vi "Micro-PL v10.2.0.vi"() -> ()   [LabVIEW 2010]
uses:
  drivers/Oxford ITC/ITCAPPS.LLB/ITCSetup.ctl
  drivers/Oxford ITC/ITCSUBS.LLB/ITCIO.ctl
  drivers/Oxford ITC/BUSGEN.LLB/OxfordAddress.ctl
  drivers/Oxford ITC/ITCSUBS.LLB/ITCVersion.ctl
  subvi/ESA-C/TypeDefs/ESA-C Live Controls.ctl
  subvi/ESA-C/TypeDefs/ESA-C Current Values.ctl
  subvi/ESA-C/TypeDefs/ESA-C Connection Settings.ctl
  subvi/ESA-C/TypeDefs/ESA-C Set Positions.ctl
  subvi/ITC503/TypeDefs/ITC503 Settings.ctl
  subvi/ITC503/TypeDefs/ITC503 Current Values.ctl
  subvi/iHR550/TypeDefs/iHR Current Values.ctl
  subvi/iHR550/TypeDefs/iHR Settings.ctl
  subvi/Mapping/TypeDefs/Mapping Spectra Params.ctl
  <vilib>/Utility/miscctls.llb/LVBoundsTypeDef.ctl
  <vilib>/Utility/miscctls.llb/LVPointTypeDef.ctl
  drivers/Horiba Spectrum One 3000V/Lib/CCD_command.llb/Comm Params.ctl
panel:
  out "ITC503 Temp Storage":dbl
  out "Runtime":u32
  out "ITC Gradient Time":i64
  out "Read ITC":bool
  out "Read CCD3500":bool
  out "Read iHR550":bool
  out "Read Drive":bool
  out "Spectrum Properties":cluster{"Position":T1, "Plot Area Size":T1}={"Position"={"Width"=36, "Height"=367}, "Plot Area Size"={"Width"=496, "Height"=264}}
  in  "Auto Folder":path caption="Ausgewählter Pfad"
  out "Int. Time Temp":dbl
  out "Wavelengths (nm)":dbl[](array[numeric])
  out "Measurement Running":bool
  out "ITC503s Running":bool
  out "Drive Running":bool
  out "CCD3500V Running":bool
  out "iHR550 Running":bool
  in  "Exit":bool
  out "iHR550 Status":bool
  out "Drive Status":bool
  out "CCD3500V Status":bool
  out "ITC503 Status":bool
  in  "CCD3500V Connection":T2={"Comm Interface"=1, "BUS"=0, "Address"=5, "Com Port"=0}
  out "Video Running":bool
  out "iHR550 RefNum":refnum<k7> caption="Mono RefNum out"
  out "ITC Setup":T3={"Description"="", "IO Info"={"Address"={"Com Port"=1, "ISOBUS Address"=1, "GPIB Address"=24, "Communication"=enum."ISOBUS"}, "Version"=enum."ITC503", "Ch 1 dec places"=1, "Ch 2 dec places"=1, "Ch 3 dec places"=1, "Ch1 Name"="", "Ch2 Name"="", "Ch3 Name"=""}}
  in  "Register":enum32{"Devices", "Acquisition / Mapping"}(tab)
  out "CCD3500 Temperature":dbl caption="Temp. (°C)" min=10.0 max=160.0 step=0.1 format="%.1f"
  in  "CCD3500V GPIB-Port":i32=5 caption="GPIB-Port" min=1 max=20 step=1 format="%#.0f"
  in  "CCD3500V Connect":bool
  out "CCD Timing":u32 caption="CCD"
  out "ITC Timing":u32 caption="ITC"
  out "Drive Timing":u32 caption="Drive"
  out "iHR550 Timing":u32 caption="iHR550"
  in  "iHR550 Force Init":bool=TRUE
  in  "iHR550 Connect":bool
  in  "iHR550 ID":string(combo)="iHR550" caption="Monochromator ID"
  out "ITC503 Current Values":T7 {"ITC503 Gradient" format="%.2f"; "ITC503 Setpoint" min=-273.0 max=300000.0 step=0.0001 format="%.1f"; "ITC503 I" format="%_1f"; "ITC503 P" format="%_1f"; "ITC503 Temperature" min=0.0 max=1645.0 step=1e-05 format="%.2f"; "ITC503 Heater" min=0.0 max=100.0 step=0.01 scale=0.0..100.0}
  in  "ITC503 Settings":T8={"ITC503 Set Setpoint"=0.0, "ITC503 Set Auto Heater"=TRUE, "ITC503 Set Auto PID"=TRUE, "P"=0.0, "I"=0.0, "D"=0.0} {"D" min=0.0 max=100.0 step=0.1 format="%.1f"; "I" min=0.0 max=100.0 step=0.1 format="%.1f"; "P" min=0.0 max=100.0 step=0.1 format="%.1f"; "ITC503 Set Setpoint" min=-273.0 max=300000.0 step=0.1 format="%.1f"}
  in  "ITC503 Configure":bool
  in  "ITC503 Connect":bool
  in  "ITC503 Selector":u16(ring) caption="Select Device" items=["ITC503s"]
  out "Drive Current Values":T9 {"Position"."Drive Z Position" min=-273.0 max=300000.0 step=0.0001 format="%.1f"; "Position"."Drive Y Position" min=-273.0 max=300000.0 step=0.0001 format="%.1f"; "Position"."Drive X Position" min=-273.0 max=300000.0 step=0.0001 format="%.1f"; "Voltages"."Drive Z Voltage" min=-273.0 max=300000.0 step=0.0001 format="%.1f"; "Voltages"."Drive Y Voltage" min=-273.0 max=300000.0 step=0.0001 format="%.1f"; "Voltages"."Drive X Voltage" min=-273.0 max=300000.0 step=0.0001 format="%.1f"}
  in  "Drive Connection":T10={"Objective GPIB-Port"=4, "Stage GPIB-Port"=4, "Drive Selector"=0, "Drive Velocity (V/s)"=5.0} {"Drive Velocity (V/s)" min=10.0 max=160.0 step=0.1 format="%.1f"; "Drive Selector" items=["Obj.", "Stage"]; "Stage GPIB-Port" min=1 max=20 step=1 format="%#.0f"; "Objective GPIB-Port" min=1 max=20 step=1 format="%#.0f"}
  in  "Drive Connect":bool
  in  "Spectrum Maximize":bool
  out "Spectrum":cluster{dbl[], dbl[]}[](graph)
  in  "CCD3000 Current Rep.":string="0/0"
  in  "Spectrum Load":bool
  in  "Spectrum Save":bool
  in  "Video Show":bool
  in  "Drive GoTo":bool caption="Objective Move Abs."
  in  "Drive New Positions":T11 {"Drive X Set" min=10.0 max=160.0 step=0.1 format="%.1f"; "Drive Z Set" min=10.0 max=160.0 step=0.1 format="%.1f"; "Drive Y Set" min=10.0 max=160.0 step=0.1 format="%.1f"}
  in  "Spectrum Autosave":bool caption="iHR550 Force Init"
  in  "CCD3500 Preview":bool
  in  "CCD3500 Acquire":bool
  in  "Spectra Settings":T12={"Integration Time"=1.0, "Repetitions"=1, "Mapping Spectra"=TRUE} caption="Mapping Spectra Settings" {"Repetitions" min=1 max=100 step=1; "Integration Time" min=0.1 max=6000.0 step=0.1 format="%.1f"}
  in  "Mapping Start":bool
  in  "iHR550 Configure":bool
  in  "iHR Settings":T13={"iHR550 Set Exit Mirror"=2, "iHR550 Set Side Exit"=0.0, "iHR550 Set Front Entrance"=0.0, "iHR550 Set Wavelength"=897.9988, "iHR550 Set Grating"=0, "iHR550 Set Grating Switch"=FALSE, "iHR550 Set Wavelength Switch"=FALSE, "iHR550 Set Mirror Switch"=FALSE, "iHR550 Set Slits Switch"=FALSE} {"iHR550 Set Grating" items=["1800"=1, "600"=2, "150"=3]; "iHR550 Set Wavelength" min=0.0 max=1500.0 step=1.0; "iHR550 Set Side Exit" min=0.0 max=2000.0 step=1.0; "iHR550 Set Exit Mirror" items=["Front"=2, "Side"=3]}
  out "iHR Current Values":T14={"iHR 550 Front Entrance"=0.0, "iHR550 Side Exit"=0.0, "iHR550 Wavelength"=897.9988, "iHR550 Exit Mirror"=2, "iHR550 Grating"="1", "Grating Index"=1} {"iHR550 Exit Mirror" items=["EntranceMirror", "ExitMirror", "Front", "Side"]}
  out "Drive Live Current Values":T9 {"Position"."Drive Z Position" min=-273.0 max=300000.0 step=0.0001 format="%.1f"; "Position"."Drive Y Position" min=-273.0 max=300000.0 step=0.0001 format="%.1f"; "Position"."Drive X Position" min=-273.0 max=300000.0 step=0.0001 format="%.1f"; "Voltages"."Drive Z Voltage" min=-273.0 max=300000.0 step=0.0001 format="%.1f"; "Voltages"."Drive Y Voltage" min=-273.0 max=300000.0 step=0.0001 format="%.1f"; "Voltages"."Drive X Voltage" min=-273.0 max=300000.0 step=0.0001 format="%.1f"}
  in  "Drive Live Controls":T15={"Snapshot"=FALSE, "Move Step"=1.0, "Move Home"=FALSE, "Move Down"=FALSE, "Move Up"=FALSE, "Move Left"=FALSE, "Move Right"=FALSE, "Move Out"=FALSE, "Move In"=FALSE} {"Move Step" min=0.0 max=30.0 step=0.1 format="%.1f"}
  # "Correlation Setup"
  # "Active"
  # "Active"
  # "ITC"
  # "iHR"
  # "Drive"
  # "CCD"
  # "Status"
  # "CCD"
  # "ITC"
  # "iHR"
  # "Drive"
  # "CCD"
  # "Timing"
  # "Monochromator"
  # "Cryostat"
  # "Drives"
  # "Drive Control"
  # "Spectrum"
  # "CCD"
  # "Mapping"
  # "Launch the Spectral Mapping VI and Raman Tool Set 2.0 in a new window."
  # "Monochromator"
  # "XY"
  # "Z"
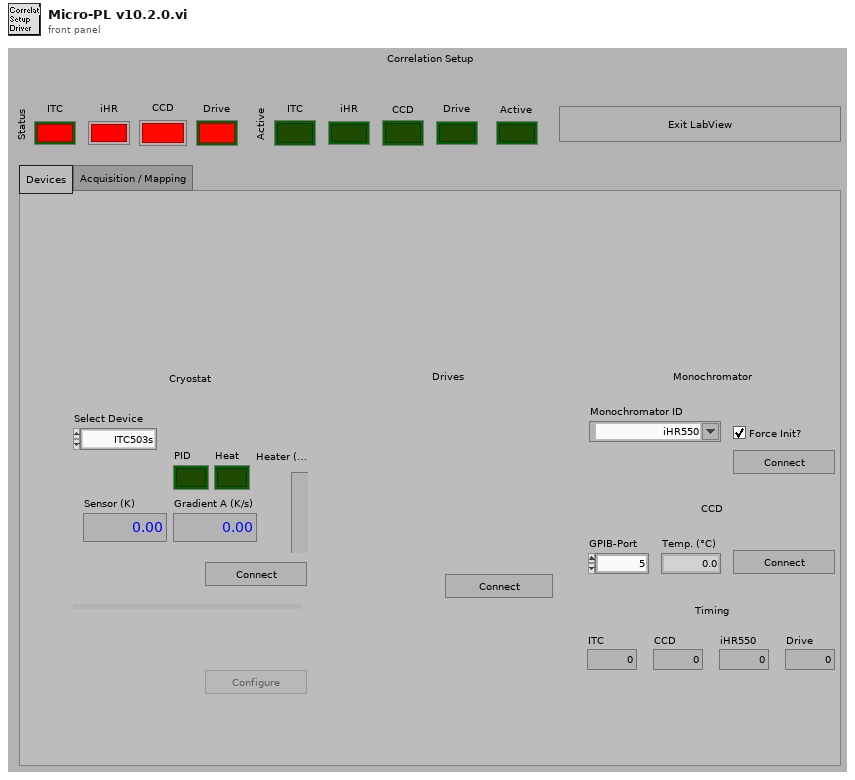
[diagram p1: front panel]
types:
  T1 = typedef "LVBoundsTypeDef.ctl" = cluster{"Width":u32, "Height":u32}
  T2 = cluster{"Comm Interface":u16, "BUS":i16, "Address":i16, "Com Port":i32}
  T3 = typedef "ITCSetup.ctl" = cluster{"Description":string, "IO Info":T4}
  T4 = typedef "ITCIO.ctl" = cluster{"Address":T5, "Version":T6, "Ch 1 dec places":i16, "Ch 2 dec places":i16, "Ch 3 dec places":i16, "Ch1 Name":string, "Ch2 Name":string, "Ch3 Name":string}
  T5 = typedef "OxfordAddress.ctl" = cluster{"Com Port":i32, "ISOBUS Address":i32, "GPIB Address":i16, "Communication":enum16{"RS232", "ISOBUS", "GPIB", "Gateway"}}
  T6 = typedef "ITCVersion.ctl" = enum16{"ITC502", "ITC503", "ITC601"}
  T7 = typedef "ITC503 Current Values.ctl" = cluster{"ITC503 Heater":dbl, "ITC503 Temperature":dbl, "ITC503 P":dbl, "ITC503 I":dbl, "ITC503 D":dbl, "ITC503 Setpoint":dbl, "ITC503 Gradient":dbl, "ITC503 Heater Auto":bool, "ITC503 PID Auto":bool}
  T8 = typedef "ITC503 Settings.ctl" = cluster{"ITC503 Set Setpoint":dbl, "ITC503 Set Auto Heater":bool, "ITC503 Set Auto PID":bool, "P":dbl, "I":dbl, "D":dbl}
  T9 = typedef "ESA-C Current Values.ctl" = cluster{"Voltages":cluster{"Drive X Voltage":dbl, "Drive Y Voltage":dbl, "Drive Z Voltage":dbl}, "Position":cluster{"Drive X Position":dbl, "Drive Y Position":dbl, "Drive Z Position":dbl}}
  T10 = typedef "ESA-C Connection Settings.ctl" = cluster{"Objective GPIB-Port":i32, "Stage GPIB-Port":i32, "Drive Selector":u16, "Drive Velocity (V/s)":dbl}
  T11 = typedef "ESA-C Set Positions.ctl" = cluster{"Drive X Set":dbl, "Drive Y Set":dbl, "Drive Z Set":dbl}
  T12 = typedef "Mapping Spectra Params.ctl" = cluster{"Integration Time":dbl, "Repetitions":u16, "Mapping Spectra":bool}
  T13 = typedef "iHR Settings.ctl" = cluster{"iHR550 Set Exit Mirror":u16, "iHR550 Set Side Exit":dbl, "iHR550 Set Front Entrance":dbl, "iHR550 Set Wavelength":dbl, "iHR550 Set Grating":u16, "iHR550 Set Grating Switch":bool, "iHR550 Set Wavelength Switch":bool, "iHR550 Set Mirror Switch":bool, "iHR550 Set Slits Switch":bool}
  T14 = typedef "iHR Current Values.ctl" = cluster{"iHR 550 Front Entrance":dbl, "iHR550 Side Exit":dbl, "iHR550 Wavelength":dbl, "iHR550 Exit Mirror":i32, "iHR550 Grating":string, "Grating Index":i32}
  T15 = typedef "ESA-C Live Controls.ctl" = cluster{"Snapshot":bool, "Move Step":dbl, "Move Home":bool, "Move Down":bool, "Move Up":bool, "Move Left":bool, "Move Right":bool, "Move Out":bool, "Move In":bool}
  T16 = typedef "LVPointTypeDef.ctl" = cluster{"Horizontal":i16, "Vertical":i16}
  T17 = enum8{"Enabled", "Disabled", "Disabled and Grayed Out"}
  T18 = typedef "Comm Params.ctl" = cluster{"Comm Interface":u16, "BUS":i16, "Address":i16, "Com Port":i32}
  T19 = enum16{"CCD Temperature Z345", "CCD Temperature Z308", "CCD Gain"}
  T20 = cluster{"CCD3000 Connection":T18, "Drive Connection Settings":T10, "ITC503 Current Values":T7, "Wavelengths (nm)":dbl[], "Drive Current Values":T9, "iHR Current Values":T14, "Spectra Settings":T12, "CCD3500 Temperature":dbl, "Simulate Drive 2":bool, "Simulate Spectra 2":bool}
  T21 = cluster{"Intensities":dbl[], "Wavelengths":dbl[]}[]
  T22 = typedef "LVPositionTypeDef.ctl" = cluster{"Left":i32, "Top":i32}
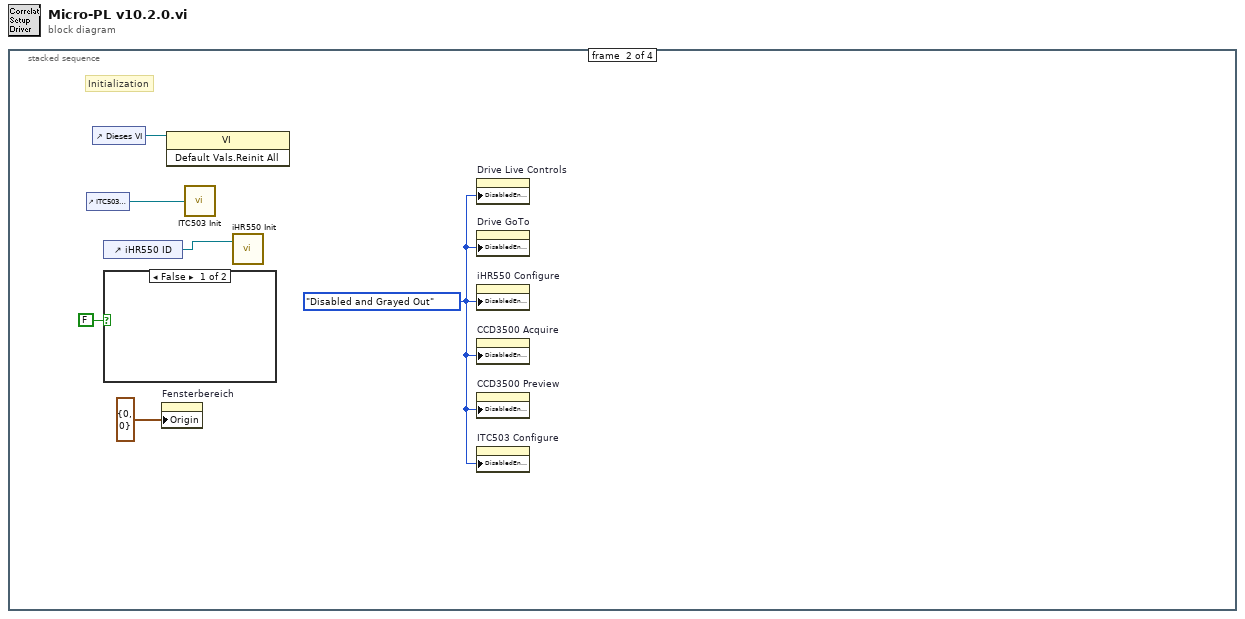
[diagram p0: block diagram]
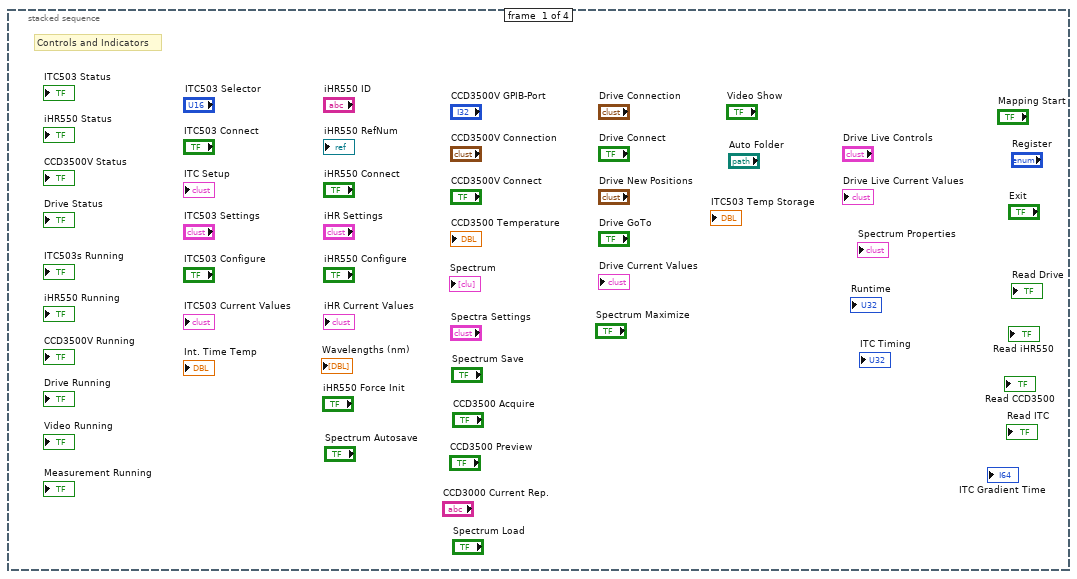
[diagram p2: hidden frame]
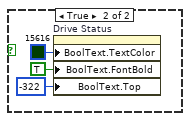
[diagram p3: hidden frame]
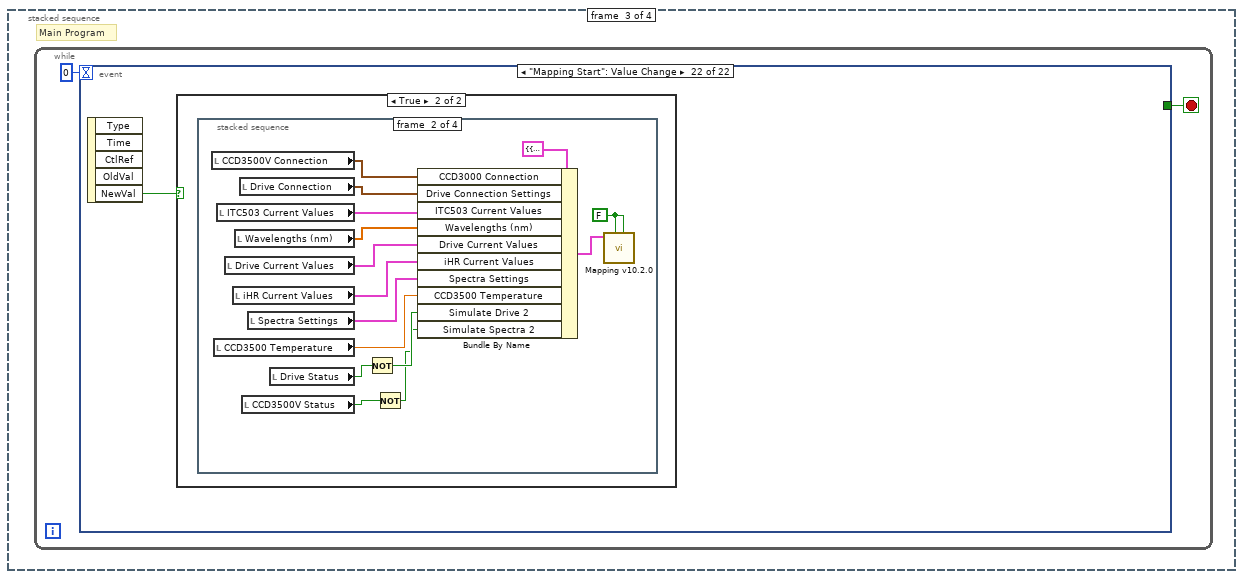
[diagram p4: hidden frame]
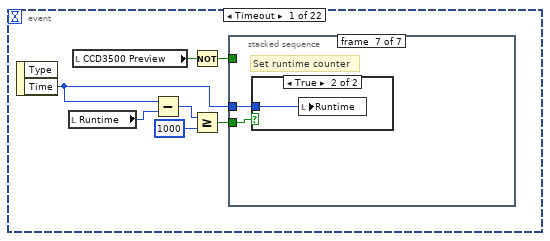
[diagram p5: hidden frame]
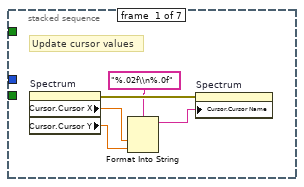
[diagram p6: hidden frame]
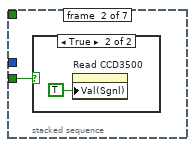
[diagram p7: hidden frame]
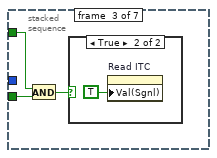
[diagram p9: hidden frame]
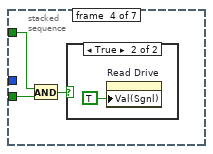
[diagram p11: hidden frame]
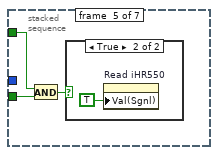
[diagram p13: hidden frame]
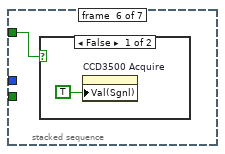
[diagram p15: hidden frame]
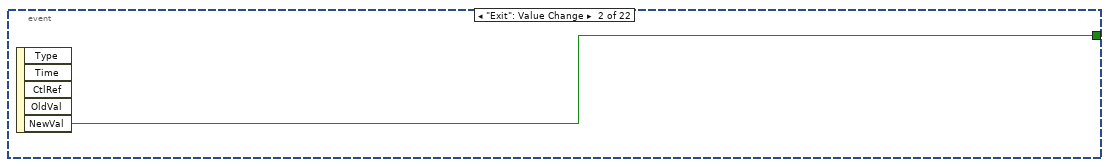
[diagram p18: hidden frame]
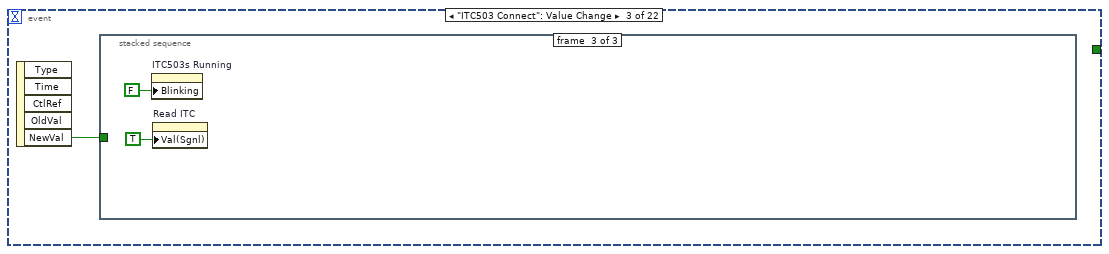
[diagram p19: hidden frame]
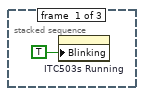
[diagram p20: hidden frame]
diagram:
  n1 = stacked-sequence {
    frame #0 {
      # "Controls and Indicators"
    }
    frame #1 {
      w1 = T17."Disabled and Grayed Out" ("Deaktiviert")
      # "Initialization"
      n2 = control-ref of="ITC503 Selector"() -> (w6:refnum<vi>)
      n3 = control-ref of="Dieses VI"() -> (w5:refnum<vi>)
      n4 = control-ref of="iHR550 ID"() -> (w4:refnum<vi>)
      n5 = case shown="False" FALSE {
        frame False {
        }
        frame True {
          n6 = property on="Drive Status" class="Bool (strict)"("BoolText.TextColor"=u32 15616, "BoolText.FontBold"=TRUE ("Boolescher Text.Schriftart:Fett"), "BoolText.Top"=-322 ("Boolescher Text.Position:Oben")) -> ()  [unwired: 2 in, 2 out]
        }
      }
      n7 = property on="Fensterbereich" class="Pane"("Origin"=T16 {"Horizontal"=0, "Vertical"=0}) -> ()  [unwired: 2 in, 2 out]
      n8 = invoke class="VI" method="Default Vals.Reinit All"(reference=w5) -> ()  [unwired: 2 in, 3 out]
      n9 = call "ITC503 Init.vi"("ITC Selector"=w6) -> ()  [unwired: 1 in]
      n10 = call "iHR550 Init.vi"("Mono ID"=w4) -> ()  [unwired: 2 in]
      n11 = property on="Drive Live Controls" class="Clust (strict)"("DisabledEnum"=w1) -> ()  [unwired: 2 in, 2 out]
      n12 = property on="Drive GoTo" class="Bool (strict)"("DisabledEnum"=w1) -> ()  [unwired: 2 in, 2 out]
      n13 = property on="iHR550 Configure" class="Bool (strict)"("DisabledEnum"=w1) -> ()  [unwired: 2 in, 2 out]
      n14 = property on="CCD3500 Acquire" class="Bool (strict)"("DisabledEnum"=w1) -> ()  [unwired: 2 in, 2 out]
      n15 = property on="CCD3500 Preview" class="Bool (strict)"("DisabledEnum"=w1) -> ()  [unwired: 2 in, 2 out]
      n16 = property on="ITC503 Configure" class="Bool (strict)"("DisabledEnum"=w1) -> ()  [unwired: 2 in, 2 out]
    }
    frame #2 {
      # "Main Program"
      n17 = while "Main-Program" {
        stop <- w11 stop-if-true
        n18 = event shown="[21] \"Mapping Start\": Value Change" {
          selector: _ -> [_ _ _ _ _ _ _ _ _ _ _ _ _ _ _ _ _ _ _ _ _ _]
          dyn-events: _ -> [_ _ _ _ _ _ _ _ _ _ _ _ _ _ _ _ _ _ _ _ _ _]
          timeout: 0 -> [_ _ _ _ _ _ _ _ _ _ _ _ _ _ _ _ _ _ _ _ _ _]
          tunnel: [_ w43 _ _ _ _ _ _ _ _ _ _ _ _ _ _ _ _ _ _ _ _] -> w11
          event Timeout {
            n19 = event-data() -> ("Time"=w13:u32)  [unwired: 1 in, 1 out]
            n20 = local read "Runtime"() -> (w12:u32)
            n21 = local read "CCD3500 Preview"() -> (w15:bool)
            n22 = Subtract(x=w13, y=w12) -> (x-y=w16:u32)
            n23 = Not(x=w15) -> (.not. x?=w14:bool)
            n24 = Greater Or Equal?(x=w16, y=u32 1000) -> (x >= y?=w17:bool)
            n25 = stacked-sequence {
              tunnel: w17 -> [_ w24 w28 w32 w36 _ w40]
              tunnel: w13 -> [_ _ _ _ _ _ w41]
              tunnel: w14 -> [_ _ w27 w31 w35 w38 _]
              frame #0 {
                # "Update cursor values"
                n26 = property on="Spectrum" class="XYGraph (strict)"() -> (error out=w23:errorcluster, "Cursor.Cursor X"=w22:dbl, "Cursor.Cursor Y"=w21:dbl)  [unwired: 2 in, 1 out]
                n27 = Format Into String(format string="%.02f\\n%.0f", w22, w21) -> (resulting string=w19:string)  [unwired: 2 in, 1 out]
                n28 = property on="Spectrum" class="XYGraph (strict)"(error in=w23, "Cursor.Cursor Name"=w19) -> ()  [unwired: 1 in, 2 out]
              }
              frame #1 {
                n29 = case shown="True" w24 {
                  frame False {
                  }
                  frame True {
                    n30 = property on="Read CCD3500" class="Bool (strict)"("Val(Sgnl)"=TRUE ("Value (Signaling)")) -> ()  [unwired: 2 in, 2 out]
                  }
                }
              }
              frame #2 {
                n31 = And(x=w27, y=w28) -> (x .and. y?=w26:bool)
                n32 = case shown="True" w26 {
                  frame False {
                  }
                  frame True {
                    n33 = property on="Read ITC" class="Bool (strict)"("Val(Sgnl)"=TRUE ("Value (Signaling)")) -> ()  [unwired: 2 in, 2 out]
                  }
                }
              }
              frame #3 {
                n34 = And(x=w31, y=w32) -> (x .and. y?=w30:bool)
                n35 = case shown="True" w30 {
                  frame False {
                  }
                  frame True {
                    n36 = property on="Read Drive" class="Bool (strict)"("Val(Sgnl)"=TRUE ("Value (Signaling)")) -> ()  [unwired: 2 in, 2 out]
                  }
                }
              }
              frame #4 {
                n37 = And(x=w35, y=w36) -> (x .and. y?=w34:bool)
                n38 = case shown="True" w34 {
                  frame False {
                  }
                  frame True {
                    n39 = property on="Read iHR550" class="Bool (strict)"("Val(Sgnl)"=TRUE ("Value (Signaling)")) -> ()  [unwired: 2 in, 2 out]
                  }
                }
              }
              frame #5 {
                n40 = case shown="False" w38 {
                  frame False {
                    n41 = property on="CCD3500 Acquire" class="Bool (strict)"("Val(Sgnl)"=TRUE ("Wert (signalisierend)")) -> ()  [unwired: 2 in, 2 out]
                  }
                  frame True {
                  }
                }
              }
              frame #6 {
                # "Set runtime counter"
                n42 = case shown="True" w40 {
                  tunnel: w41 -> [_ w42]
                  frame False {
                  }
                  frame True {
                    n43 = local write "Runtime"(w42) -> ()
                  }
                }
              }
            }
          }
          event "Exit": Value Change {
            n44 = event-data() -> ("NewVal"=w43:bool)  [unwired: 1 in, 4 out]
          }
          event "ITC503 Connect": Value Change {
            n45 = event-data() -> ("NewVal"=w44:bool)  [unwired: 1 in, 4 out]
            n46 = stacked-sequence {
              tunnel: w44 -> [_ w46 _]
              frame #0 {
                n47 = property on="ITC503s Running" class="Bool (strict)"("Blinking"=TRUE ("Blinkend")) -> ()  [unwired: 2 in, 2 out]
              }
              frame #1 {
                n48 = case shown="True" w46 {
                  selector: w46 -> [w51 _]
                  tunnel: [w51 w58] -> w48
                  frame False {
                    # "disconnect"
                    n49 = control-ref of="ITC503s Running"() -> (w52:refnum<vi>)
                    n50 = property class="Bool (strict)"(reference=w52, "Blinking"=w51, "Value"=w51) -> ()  [unwired: 1 in, 2 out]
                  }
                  frame True {
                    # "connect"
                    n51 = local read "ITC503 Selector"() -> (w59:u16)
                    n52 = call "ITC503 Connect.vi"("ITC Selector"=w59) -> ("ITC Setup"=w57:T3, "Connected"=w58:bool)
                    n53 = local write "ITC Setup"(w57) -> ()
                    n54 = call "ITC503 Get Values.vi"("ITC Setup"=w57) -> ("ITC503 Current Values"=w56:T7)  [unwired: 1 in, 1 out]
                    n55 = Unbundle By Name(w56) -> ("ITC503 Setpoint"=w53:dbl)
                    n56 = Bundle By Name(cluster=T8 {"ITC503 Set Setpoint"=0.0, "ITC503 Set Auto Heater"=TRUE, "ITC503 Set Auto PID"=TRUE, "P"=0.0, "I"=0.0, "D"=0.0} ("ITC503 Settings"), "ITC503 Set Setpoint"=w53) -> (w54:T8)
                    n57 = local write "ITC503 Settings"(w54) -> ()
                  }
                }
                n58 = case shown="False" w48 {
                  tunnel: [T17."Disabled and Grayed Out" ("Deaktiviert") T17."Enabled" ("Deaktiviert")] -> w47
                  frame False {
                  }
                  frame True {
                  }
                }
                n59 = local write "ITC503 Status"(w48) -> ()
                n60 = local write "ITC503 Connect"(w48) -> ()
                n61 = property on="ITC503 Configure" class="Bool (strict)"("DisabledEnum"=w47) -> ()  [unwired: 2 in, 2 out]
              }
              frame #2 {
                n62 = property on="ITC503s Running" class="Bool (strict)"("Blinking"=FALSE ("Blinkend")) -> ()  [unwired: 2 in, 2 out]
                n63 = property on="Read ITC" class="Bool (strict)"("Val(Sgnl)"=TRUE ("Wert (signalisierend)")) -> ()  [unwired: 2 in, 2 out]
              }
            }
          }
          event "Read ITC": Value Change {
            n64 = event-data() -> ("Time"=w63:u32, "NewVal"=w67:bool)  [unwired: 1 in, 3 out]
            n65 = local read "ITC503 Status"() -> (w66:bool)
            n66 = control-ref of="ITC503s Running"() -> (w64:refnum<vi>)
            n67 = And(x=w66, y=w67) -> (x .and. y?=w65:bool)
            n68 = case shown="True" w65 {
              tunnel: w64 -> [w69 w73]
              tunnel: w63 -> [_ w72]
              tunnel: [u32 0 w71] -> w62
              frame False {
                n69 = property class="Bool (strict)"(reference=w69, "BoolText.Text"="" ("Boolescher Text.Text")) -> ()  [unwired: 1 in, 2 out]
              }
              frame True {
                n70 = stacked-sequence {
                  seq-local: [_ w78 _ _] -> [_ _ w95 _]
                  seq-local: [w74 _ _ _] -> [_ _ _ w101]
                  tunnel: w73 -> [_ _ w88 _]
                  tunnel: w72 -> [_ w79 _ _]
                  tunnel: [_ _ _ w102] -> w71
                  frame #0 {
                    n71 = Tick Count (ms)() -> (millisecond timer value=w74:u32)
                  }
                  frame #1 {
                    n72 = local read "ITC Setup"() -> (w86:T3)
                    n73 = local read "ITC Gradient Time"() -> (w83:i64)
                    n74 = call "ITC503 Get Values.vi"("ITC Setup"=w86) -> ("ITC503 Current Values"=w78:T7)  [unwired: 1 in, 1 out]
                    n75 = local read "ITC503 Temp Storage"() -> (w77:dbl)
                    n76 = Unbundle By Name(w78) -> ("ITC503 Temperature"=w75:dbl)
                    n77 = Subtract(x=w79, y=w83) -> (x-y=w82:i64)
                    n78 = Divide(x=w82, y=i64 1000) -> (x/y=w80:dbl)
                    n79 = Subtract(x=w75, y=w77) -> (x-y=w76:dbl)
                    n80 = Divide(x=w76, y=w80) -> (x/y=w85:dbl)
                    n81 = Bundle By Name(cluster=w78, "ITC503 Gradient"=w85) -> (w84:T7)
                    n82 = local write "ITC503 Current Values"(w84) -> ()
                  }
                  frame #2 {
                    n83 = Unbundle By Name(w95) -> ("ITC503 Temperature"=w87:dbl, "ITC503 Setpoint"=w96:dbl)
                    n84 = Subtract(x=w87, y=w96) -> (x-y=w97:dbl)
                    n85 = Number To Fractional String(number=w87, precision (6)=i16 2 ("Genauigkeit (6)")) -> (F-format string=w91:string)  [unwired: 2 in]
                    n86 = Absolute Value(x=w97) -> (abs(x)=w98:dbl)
                    n87 = String Subset(string=w91, length (rest)=5 ("Länge (Rest)")) -> (substring=w89:string)  [unwired: 1 in]
                    n88 = Greater?(x=w98, y=2.0) -> (0:w94:bool)
                    n89 = Not(x=w94) -> (.not. x?=w93:bool)
                    n90 = property class="Bool (strict)"(reference=w88, "Blinking"=w94, "Value"=w93, "BoolText.Text"=w89) -> ()  [unwired: 1 in, 2 out]
                    n91 = local write "ITC503 Temp Storage"(w87) -> ()
                  }
                  frame #3 {
                    n92 = Tick Count (ms)() -> (millisecond timer value=w100:u32)
                    n93 = local write "ITC Gradient Time"(w100) -> ()
                    n94 = Subtract(x=w100, y=w101) -> (x-y=w102:u32)
                  }
                }
              }
            }
            n95 = local write "ITC Timing"(w62) -> ()
          }
          event "iHR550 Connect": Value Change {
            n96 = event-data() -> ("NewVal"=w103:bool)  [unwired: 1 in, 4 out]
            n97 = stacked-sequence {
              tunnel: w103 -> [_ w106 _]
              frame #0 {
                n98 = property on="iHR550 Running" class="Bool (strict)"("Blinking"=TRUE ("Blinkend")) -> ()  [unwired: 2 in, 2 out]
              }
              frame #1 {
                n99 = case shown="True" w106 {
                  selector: w106 -> [w110 _]
                  tunnel: [w110 w123] -> w105
                  frame False {
                    # "disconnect"
                  }
                  frame True {
                    # "connect"
                    n100 = local read "iHR550 Force Init"() -> (w121:bool)
                    n101 = control-ref of="iHR550 Set Grating"() -> (w122:refnum<vi>)
                    n102 = local read "iHR550 ID"() -> (w124:string)
                    n103 = call "iHR550 Connect.vi"("Force\nInitialization"=w121, "Grating Selector"=w122, "Mono ID"=w124) -> ("Initialized"=w123:bool, "iHR550 RefNum"=w120:refnum<k7>)  [unwired: 2 in, 4 out]
                    n104 = local write "iHR550 RefNum"(w120) -> ()
                    n105 = call "iHR550 Read Values.vi"("JYMONOLib.IJYMonoReqd"=w120) -> ("iHR Current Values"=w112:T14)  [unwired: 1 in]
                    n106 = local write "iHR Current Values"(w112) -> ()
                    n107 = Unbundle By Name(w112) -> ("iHR 550 Front Entrance"=w118:dbl, "iHR550 Side Exit"=w117:dbl, "iHR550 Wavelength"=w116:dbl, "iHR550 Exit Mirror"=w115:i32, "Grating Index"=w113:i32)
                    n108 = call "iHR550 Convert Axis.vi"("iHR Current Values"=w112) -> ("Wavelengths (nm)"=w111:dbl[])
                    n109 = local write "Wavelengths (nm)"(w111) -> ()
                    n110 = Bundle By Name(cluster=T13 {"iHR550 Set Exit Mirror"=0, "iHR550 Set Side Exit"=0.0, "iHR550 Set Front Entrance"=0.0, "iHR550 Set Wavelength"=0.0, "iHR550 Set Grating"=0, "iHR550 Set Grating Switch"=FALSE, "iHR550 Set Wavelength Switch"=FALSE, "iHR550 Set Mirror Switch"=FALSE, "iHR550 Set Slits Switch"=FALSE} ("iHR Settings"), "iHR550 Set Front Entrance"=w118, "iHR550 Set Side Exit"=w117, "iHR550 Set Wavelength"=w116, "iHR550 Set Exit Mirror"=w115, "iHR550 Set Grating"=w113) -> (w114:T13)
                    n111 = local write "iHR Settings"(w114) -> ()
                  }
                }
                n112 = local write "iHR550 Status"(w105) -> ()
                n113 = local write "iHR550 Connect"(w105) -> ()
                n114 = case shown="False" w105 {
                  tunnel: [T17."Disabled and Grayed Out" ("Deaktiviert") T17."Enabled" ("Deaktiviert")] -> w107
                  frame False {
                  }
                  frame True {
                  }
                }
                n115 = property on="iHR550 Configure" class="Bool (strict)"("DisabledEnum"=w107) -> ()  [unwired: 2 in, 2 out]
              }
              frame #2 {
                n116 = local write "iHR550 Force Init"(FALSE ("iHR550 Force Init")) -> ()
                n117 = property on="iHR550 Running" class="Bool (strict)"("Blinking"=FALSE ("Blinkend")) -> ()  [unwired: 2 in, 2 out]
                n118 = property on="Read iHR550" class="Bool (strict)"("Val(Sgnl)"=TRUE ("Wert (signalisierend)")) -> ()  [unwired: 2 in, 2 out]
              }
            }
          }
          event "Read iHR550": Value Change {
            n119 = event-data() -> ("NewVal"=w131:bool)  [unwired: 1 in, 4 out]
            n120 = local read "iHR550 Status"() -> (w130:bool)
            n121 = And(x=w130, y=w131) -> (x .and. y?=w129:bool)
            n122 = case shown="False" w129 {
              tunnel: [u32 0 w133] -> w128
              frame False {
              }
              frame True {
                n123 = stacked-sequence {
                  seq-local: [w134 _ _] -> [_ _ w137]
                  tunnel: [_ _ w138] -> w133
                  frame #0 {
                    n124 = Tick Count (ms)() -> (millisecond timer value=w134:u32)
                  }
                  frame #1 {
                    n125 = local read "iHR550 RefNum"() -> (w136:refnum<k7>)
                    n126 = call "iHR550 Read Values.vi"("JYMONOLib.IJYMonoReqd"=w136) -> ("iHR Current Values"=w135:T14)  [unwired: 1 in]
                    n127 = local write "iHR Current Values"(w135) -> ()
                  }
                  frame #2 {
                    n128 = Tick Count (ms)() -> (millisecond timer value=w139:u32)
                    n129 = Subtract(x=w139, y=w137) -> (x-y=w138:u32)
                  }
                }
              }
            }
            "iHR550 Timing" <- w128
          }
          event "CCD3500V Connect": Value Change {
            n130 = event-data() -> ("NewVal"=w140:bool)  [unwired: 1 in, 4 out]
            n131 = stacked-sequence {
              tunnel: w140 -> [_ w142 _]
              frame #0 {
                n132 = property on="CCD3500V Running" class="Bool (strict)"("Blinking"=TRUE ("Blinkend")) -> ()  [unwired: 2 in, 2 out]
              }
              frame #1 {
                n133 = case shown="True" w142 {
                  selector: w142 -> [w148 _]
                  tunnel: [w148 w149] -> w144
                  frame False {
                    # "disconnect"
                    n134 = local read "CCD3500V Connection"() -> (w147:T2)
                    n135 = call "CCDSTOP.VI"("Comm Params"=w147) -> ()  [unwired: 1 out]
                  }
                  frame True {
                    # "connect"
                    n136 = stacked-sequence {
                      seq-local: [_ w153 _] -> [_ _ w155]
                      tunnel: [_ w154 _] -> w149
                      frame #0 {
                        n137 = local read "CCD3500V GPIB-Port"() -> (w151:i32)
                        n138 = Bundle By Name(cluster=T18 {"Comm Interface"=1, "BUS"=0, "Address"=5, "Com Port"=1} ("Comm Params"), "Address"=w151) -> (w152:T18)
                        n139 = local write "CCD3500V Connection"(w152) -> ()
                      }
                      frame #1 {
                        n140 = local read "CCD3500V Connection"() -> (w153:T2)
                        n141 = call "CCD3000 Initialize.vi"("Comm Params"=w153) -> ("Success"=w154:bool)  [unwired: 9 in, 1 out]
                      }
                      frame #2 {
                        n142 = local read "Spectra Settings"() -> (w156:T12)
                        n143 = Unbundle By Name(w156) -> ("Integration Time"=w157:dbl)
                        n144 = local write "Int. Time Temp"(w157) -> ()
                        n145 = call "CCD3000 Prepare Acquisition.vi"("Mapping Spectra Settings"=w156, "Comm Params"=w155) -> ()  [unwired: 4 in]
                      }
                    }
                  }
                }
                n146 = local write "CCD3500V Connect"(w144) -> ()
                n147 = local write "CCD3500V Status"(w144) -> ()
                n148 = case shown="False" w144 {
                  tunnel: [T17."Disabled and Grayed Out" ("Deaktiviert") T17."Enabled" ("Deaktiviert")] -> w143
                  frame False {
                  }
                  frame True {
                  }
                }
                n149 = property on="CCD3500V Status" class="Bool (strict)"("BoolText.Visible"=w144) -> ()  [unwired: 2 in, 2 out]
                n150 = property on="CCD3500 Acquire" class="Bool (strict)"("DisabledEnum"=w143) -> ()  [unwired: 2 in, 2 out]
                n151 = property on="CCD3500 Preview" class="Bool (strict)"("DisabledEnum"=w143) -> ()  [unwired: 2 in, 2 out]
              }
              frame #2 {
                n152 = property on="Read CCD3500" class="Bool (strict)"("Val(Sgnl)"=TRUE ("Wert (signalisierend)")) -> ()  [unwired: 2 in, 2 out]
                n153 = property on="CCD3500V Running" class="Bool (strict)"("Blinking"=FALSE ("Blinkend")) -> ()  [unwired: 2 in, 2 out]
              }
            }
          }
          event "Read CCD3500": Value Change {
            n154 = event-data() -> ("NewVal"=w163:bool)  [unwired: 1 in, 4 out]
            n155 = local read "CCD3500V Status"() -> (w162:bool)
            n156 = And(x=w162, y=w163) -> (x .and. y?=w161:bool)
            n157 = case shown="False" w161 {
              tunnel: [u32 0 w165] -> w160
              frame False {
              }
              frame True {
                n158 = stacked-sequence {
                  seq-local: [_ w167 _ _] -> [_ _ w176 _]
                  seq-local: [w166 _ _ _] -> [_ _ _ w183]
                  tunnel: [_ _ _ w184] -> w165
                  frame #0 {
                    n159 = Tick Count (ms)() -> (millisecond timer value=w166:u32)
                  }
                  frame #1 {
                    n160 = local read "CCD3500V Connection"() -> (w171:T2)
                    n161 = call "PROPGET.VI"("CCD Prop ID"=T19."CCD Temperature Z345", "Comm Params"=w171) -> ("Output Param"=w169:dbl)  [unwired: 1 out]
                    n162 = Subtract(x=w169, y=273.15) -> (x-y=w167:dbl)
                    n163 = local write "CCD3500 Temperature"(w167) -> ()
                  }
                  frame #2 {
                    n164 = Greater?(x=w176, y=-115.0) -> (0:w172:bool)
                    n165 = case shown="True" w172 {
                      selector: w172 -> [w180 w182]
                      tunnel: [cluster{u32, u32}[] [{16713728, 16713728}, {6618880, 6618880}] ("Farben [4]") cluster{u32, u32}[] [{16713728, 16713728}] ("Farben [4]")] -> w173
                      tunnel: [w180 w182] -> w175
                      frame False {
                      }
                      frame True {
                      }
                    }
                    n166 = Number To Fractional String(number=w176, precision (6)=i16 1 ("Genauigkeit (6)")) -> (F-format string=w174:string)  [unwired: 2 in]
                    n167 = property on="CCD3500V Status" class="Bool (strict)"("Blinking"=w175, "BoolText.Text"=w174, "Colors [4]"=w173) -> ()  [unwired: 2 in, 2 out]
                  }
                  frame #3 {
                    n168 = Tick Count (ms)() -> (millisecond timer value=w185:u32)
                    n169 = Subtract(x=w185, y=w183) -> (x-y=w184:u32)
                  }
                }
              }
            }
            "CCD Timing" <- w160
          }
          event "Drive Connect": Value Change {
            n170 = event-data() -> ("NewVal"=w186:bool)  [unwired: 1 in, 4 out]
            n171 = stacked-sequence {
              tunnel: w186 -> [_ w190 _]
              frame #0 {
                n172 = property on="Drive Running" class="Bool (strict)"("Blinking"=TRUE ("Blinkend")) -> ()  [unwired: 2 in, 2 out]
              }
              frame #1 {
                n173 = local read "Drive Connection"() -> (w191:T10)
                n174 = Not(x=w190) -> (.not. x?=w192:bool)
                n175 = call "ESA-C Connect.vi"("Remote=F /Local=T"=w192, "Drive Connection Settings"=w191) -> ("Success"=w193:bool)  [unwired: 2 in]
                n176 = Exclusive Or(1:w192, 2:w193) -> (0:w194:bool)
                n177 = local write "Drive Connect"(w194) -> ()
                n178 = local write "Drive Status"(w194) -> ()
                n179 = case shown="False" w194 {
                  tunnel: [T17."Disabled and Grayed Out" ("Deaktiviert") T17."Enabled" ("Deaktiviert")] -> w189
                  tunnel: ["" ("Boolescher Text.Text") w197] -> w188
                  frame False {
                  }
                  frame True {
                    n180 = property on="Drive Selector" class="Ring (strict)"() -> ("RingText.Text"=w197:string)  [unwired: 2 in, 2 out]
                  }
                }
                n181 = property on="Drive Live Controls" class="Clust (strict)"("DisabledEnum"=w189) -> ()  [unwired: 2 in, 2 out]
                n182 = property on="Drive Status" class="Bool (strict)"("BoolText.Text"=w188) -> ()  [unwired: 2 in, 2 out]
                n183 = property on="Drive GoTo" class="Bool (strict)"("DisabledEnum"=w189) -> ()  [unwired: 2 in, 2 out]
              }
              frame #2 {
                n184 = property on="Drive Running" class="Bool (strict)"("Blinking"=FALSE ("Blinkend")) -> ()  [unwired: 2 in, 2 out]
                n185 = property on="Read Drive" class="Bool (strict)"("Val(Sgnl)"=TRUE ("Wert (signalisierend)")) -> ()  [unwired: 2 in, 2 out]
              }
            }
          }
          event "Read Drive": Value Change {
            n186 = event-data() -> ("NewVal"=w204:bool)  [unwired: 1 in, 4 out]
            n187 = local read "Drive Status"() -> (w203:bool)
            n188 = And(x=w203, y=w204) -> (x .and. y?=w202:bool)
            n189 = case shown="False" w202 {
              tunnel: [u32 0 w206] -> w201
              frame False {
              }
              frame True {
                n190 = stacked-sequence {
                  seq-local: [w207 _ _] -> [_ _ w211]
                  tunnel: [_ _ w210] -> w206
                  frame #0 {
                    n191 = Tick Count (ms)() -> (millisecond timer value=w207:u32)
                  }
                  frame #1 {
                    n192 = local read "Drive Connection"() -> (w208:T10)
                    n193 = call "ESA-C Get Values.vi"("Drive Connection Settings"=w208) -> ("Drive Current Values"=w209:T9)
                    n194 = local write "Drive Live Current Values"(w209) -> ()
                    n195 = local write "Drive Current Values"(w209) -> ()
                  }
                  frame #2 {
                    n196 = Tick Count (ms)() -> (millisecond timer value=w212:u32)
                    n197 = Subtract(x=w212, y=w211) -> (x-y=w210:u32)
                  }
                }
              }
            }
            "Drive Timing" <- w201
          }
          event "Video Show": Value Change {
            n198 = event-data() -> ("NewVal"=w213:bool)  [unwired: 1 in, 4 out]
            n199 = case shown="False" w213 {
              frame False {
                n200 = call "Video Close.vi"() -> ()  [unwired: 11 in, 1 out]
              }
              frame True {
                n201 = call "Video Open.vi"() -> ()  [unwired: 11 in, 1 out]
              }
            }
          }
          event "ITC503 Configure": Value Change {
            n202 = event-data() -> ("NewVal"=w214:bool)  [unwired: 1 in, 4 out]
            n203 = stacked-sequence {
              tunnel: w214 -> [_ w216 _]
              frame #0 {
                n204 = property on="ITC503s Running" class="Bool (strict)"("Blinking"=TRUE ("Blinkend")) -> ()  [unwired: 2 in, 2 out]
              }
              frame #1 {
                n205 = local read "ITC503 Status"() -> (w218:bool)
                n206 = And(x=w218, y=w216) -> (x .and. y?=w217:bool)
                n207 = case shown="True" w217 {
                  frame False {
                  }
                  frame True {
                    n208 = local read "ITC503 Settings"() -> (w219:T8)
                    n209 = local read "ITC Setup"() -> (w220:T3)
                    n210 = call "ITC503 Set Values.vi"("Set Channel"=i16 1, "ITC503 Settings"=w219, "ITC Setup"=w220) -> ()  [unwired: 2 in]
                  }
                }
              }
              frame #2 {
                w223 = FALSE ("Blinkend")
                n211 = local write "ITC503 Configure"(w223) -> ()
                n212 = property on="ITC503s Running" class="Bool (strict)"("Blinking"=w223) -> ()  [unwired: 2 in, 2 out]
                n213 = property on="Read ITC" class="Bool (strict)"("Val(Sgnl)"=TRUE ("Wert (signalisierend)")) -> ()  [unwired: 2 in, 2 out]
              }
            }
          }
          event "iHR550 Configure": Value Change {
            n214 = event-data() -> ("NewVal"=w224:bool)  [unwired: 1 in, 4 out]
            n215 = stacked-sequence {
              tunnel: w224 -> [_ w226 _]
              frame #0 {
                n216 = property on="iHR550 Running" class="Bool (strict)"("Blinking"=TRUE ("Blinkend")) -> ()  [unwired: 2 in, 2 out]
              }
              frame #1 {
                n217 = local read "iHR550 Status"() -> (w228:bool)
                n218 = local read "iHR550 RefNum"() -> (w229:refnum<k7>)
                n219 = And(x=w228, y=w226) -> (x .and. y?=w227:bool)
                n220 = case shown="True" w227 {
                  tunnel: w229 -> [_ w230]
                  frame False {
                  }
                  frame True {
                    n221 = stacked-sequence {
                      seq-local: [_ w235 _] -> [_ _ w238]
                      tunnel: w230 -> [w231 w236 _]
                      frame #0 {
                        w234 = u16 2 items=["Front"=2, "Side"=3] ("Entrance Mirror")
                        n222 = local read "iHR Settings"() -> (w232:T13)
                        n223 = call "iHR550 Set Values.vi"("Refnum out"=w231, "Entrance Mirror"=w234, "Target\nSide Entrance"=0.0 ("Target\nSide Entrance"), "iHR Settings"=w232) -> ()  [unwired: 11 in, 1 out]
                      }
                      frame #1 {
                        n224 = call "iHR550 Read Values.vi"("JYMONOLib.IJYMonoReqd"=w236) -> ("iHR Current Values"=w235:T14)  [unwired: 1 in]
                        n225 = local write "iHR Current Values"(w235) -> ()
                      }
                      frame #2 {
                        n226 = call "iHR550 Convert Axis.vi"("iHR Current Values"=w238) -> ("Wavelengths (nm)"=w237:dbl[])
                        n227 = local write "Wavelengths (nm)"(w237) -> ()
                      }
                    }
                  }
                }
              }
              frame #2 {
                w240 = FALSE ("Blinkend")
                n228 = property on="Read iHR550" class="Bool (strict)"("Val(Sgnl)"=TRUE ("Wert (signalisierend)")) -> ()  [unwired: 2 in, 2 out]
                n229 = local write "iHR550 Configure"(w240) -> ()
                n230 = property on="iHR550 Running" class="Bool (strict)"("Blinking"=w240) -> ()  [unwired: 2 in, 2 out]
              }
            }
          }
          event "CCD3500 Preview": Value Change {
            n231 = event-data() -> ("NewVal"=w241:bool)  [unwired: 1 in, 4 out]
            n232 = case shown="True" w241 {
              frame False {
              }
              frame True {
                n233 = property on="CCD3500 Acquire" class="Bool (strict)"("Val(Sgnl)"=TRUE ("Wert (signalisierend)")) -> ()  [unwired: 2 in, 2 out]
              }
            }
          }
          event "CCD3500 Acquire": Value Change {
            n234 = event-data() -> ("NewVal"=w243:bool)  [unwired: 1 in, 4 out]
            n235 = stacked-sequence {
              tunnel: w243 -> [w244 _]
              frame #0 {
                n236 = case shown="True" w244 {
                  frame False {
                  }
                  frame True {
                    n237 = local read "CCD3500V Connection"() -> (w245:T2)
                    n238 = local read "Spectra Settings"() -> (w246:T12)
                    n239 = stacked-sequence {
                      tunnel: w246 -> [w249 w261 _]
                      tunnel: w245 -> [w248 w257 _]
                      frame #0 {
                        # "prepare acquisition if settings changed"
                        n240 = Unbundle By Name(w249) -> ("Integration Time"=w247:dbl)
                        n241 = local read "Int. Time Temp"() -> (w250:dbl)
                        n242 = Equal?(x=w247, y=w250) -> (x = y?=w251:bool)
                        n243 = case shown="False" w251 {
                          tunnel: w250 -> [_ _]
                          tunnel: w249 -> [w254 _]
                          tunnel: w248 -> [w253 _]
                          tunnel: w247 -> [w252 _]
                          frame False {
                            n244 = local write "Int. Time Temp"(w252) -> ()
                            n245 = call "CCD3000 Prepare Acquisition.vi"("Mapping Spectra Settings"=w254, "Comm Params"=w253) -> ()  [unwired: 4 in]
                          }
                          frame True {
                          }
                        }
                      }
                      frame #1 {
                        n246 = local read "CCD3500 Preview"() -> (w260:bool)
                        n247 = Unbundle By Name(w261) -> ("Repetitions"=w258:u16)
                        n248 = Select(t=i8 1, s=w260, f=w258) -> (s? t:f=w256:u16)
                        n249 = for {
                          N: w256 -> [w266]
                          tunnel: w257 -> [w278]
                          shift-right: [w273] -> _
                          shift-left: u16[][] [] -> [w276]
                          i -> [w267]
                          stop <- w272 continue-if-true
                          n250 = control-ref of="CCD3500 Acquire"() -> (w271:refnum<vi>)
                          n251 = control-ref of="CCD3500V Running"() -> (w270:refnum<vi>)
                          n252 = call "CCD3000 Spectral Acquisition.vi"("Acquire"=w271, "Running"=w270, "Comm Params"=w278) -> ("Raw-Spectrum"=w277:u16[])  [unwired: 6 in, 2 out]
                          n253 = Number To Decimal String(number=w266) -> (decimal integer string=w265:string)  [unwired: 1 in]
                          n254 = Build Array (concatenate)(w277, w276) -> (w273:u16[][])
                          n255 = Increment(x=w267) -> (x+1=w263:i32)
                          n256 = Number To Decimal String(number=w263) -> (decimal integer string=w264:string)  [unwired: 1 in]
                          n257 = local read "Wavelengths (nm)"() -> (w275:dbl[])
                          n258 = Concatenate Strings(w264, "/" ("string"), w265) -> (w269:string)
                          n259 = call "CCD3000 Average Spectra.vi"("Repetitions"=w263, "Raw Spectra"=w273) -> ("Raw Spectrum"=w274:dbl[])
                          n260 = local read "CCD3500 Acquire"() -> (w272:bool)
                          n261 = local write "CCD3000 Current Rep."(w269) -> ()
                          n262 = call "CCD3000 Pixel to Wavelength v10.1.0.vi"("Wavelengths (nm)"=w275, "Raw Spectrum"=w274) -> ("Spectrum-Cluster"=w262:T21)  [unwired: 1 out]
                          n263 = local write "Spectrum"(w262) -> ()
                        }
                      }
                      frame #2 {
                        n264 = local read "Spectrum Autosave"() -> (w279:bool)
                        n265 = case shown="True" w279 {
                          frame False {
                          }
                          frame True {
                            n266 = property on="Spectrum Save" class="Bool (strict)"("Val(Sgnl)"=TRUE ("Value (Signaling)")) -> ()  [unwired: 2 in, 2 out]
                          }
                        }
                      }
                    }
                  }
                }
              }
              frame #1 {
                n267 = local write "CCD3500 Acquire"(FALSE ("Blinkend")) -> ()
                n268 = local write "CCD3000 Current Rep."("0/0" ("CCD3000 Current Rep.")) -> ()
              }
            }
          }
          event "Drive GoTo": Value Change {
            n269 = event-data() -> ("NewVal"=w283:bool)  [unwired: 1 in, 4 out]
            n270 = stacked-sequence {
              tunnel: w283 -> [_ w285 _]
              frame #0 {
                n271 = property on="Drive Running" class="Bool (strict)"("Blinking"=TRUE ("Blinkend")) -> ()  [unwired: 2 in, 2 out]
              }
              frame #1 {
                n272 = local read "Drive Status"() -> (w287:bool)
                n273 = And(x=w287, y=w285) -> (x .and. y?=w286:bool)
                n274 = case shown="True" w286 {
                  frame False {
                  }
                  frame True {
                    n275 = local read "Drive New Positions"() -> (w288:T11)
                    n276 = local read "Drive Connection"() -> (w289:T10)
                    n277 = control-ref of="Drive Running"() -> (w290:refnum<vi>)
                    n278 = call "ESA-C Move Absolute.vi"("Running"=w290, "Drive New Abs. Positions"=w288, "Drive Connection Settings"=w289) -> ()  [unwired: 2 in]
                  }
                }
              }
              frame #2 {
                w292 = FALSE ("Blinkend")
                n279 = local write "Drive GoTo"(w292) -> ()
                n280 = property on="Drive Running" class="Bool (strict)"("Blinking"=w292) -> ()  [unwired: 2 in, 2 out]
                n281 = property on="Read Drive" class="Bool (strict)"("Val(Sgnl)"=TRUE ("Wert (signalisierend)")) -> ()  [unwired: 2 in, 2 out]
              }
            }
          }
          event Value Change {
            n282 = event-data() -> ("NewVal"=w294:bool)  [unwired: 1 in, 4 out]
            n283 = local read "Drive Status"() -> (w295:bool)
            n284 = And(x=w295, y=w294) -> (x .and. y?=w293:bool)
            n285 = case shown="True" w293 {
              frame False {
              }
              frame True {
                n286 = stacked-sequence {
                  seq-local: [w296 _ _] -> [_ w317 _]
                  frame #0 {
                    # "Move and Read"
                    n287 = flat-sequence {
                      tunnel: [w305] -> w301
                      tunnel: [w303] -> w300
                      tunnel: [w302] -> w299
                      tunnel: w301 -> [w307]
                      tunnel: w300 -> [w309]
                      tunnel: [w309] -> w298
                      tunnel: w299 -> [w308]
                      tunnel: [w306] -> w297
                      tunnel: w298 -> [w316]
                      tunnel: w297 -> [w314]
                      tunnel: [w314] -> w296
                      frame #0 {
                        n288 = local read "Drive Live Controls"() -> (w302:T15)
                        n289 = local read "Drive Connection"() -> (w303:T10)
                        n290 = control-ref of="Drive Running"() -> (w304:refnum<vi>)
                        n291 = call "ESA-C Live Control.vi"("Running"=w304, "Drive Live Controls"=w302, "Drive Connection Settings"=w303) -> ("Reset Switches"=w305:bool)  [unwired: 1 in]
                      }
                      frame #1 {
                        n292 = case shown="True" w307 {
                          tunnel: w308 -> [w310 w313]
                          tunnel: [w310 w312] -> w306
                          frame False {
                          }
                          frame True {
                            w311 = FALSE ("Move Out")
                            n293 = Bundle By Name(cluster=w313, "Move Home"=w311, "Move Down"=w311, "Move Up"=w311, "Move Left"=w311, "Move Right"=w311, "Move Out"=w311, "Move In"=w311) -> (w312:T15)
                          }
                        }
                      }
                      frame #2 {
                        n294 = local write "Drive Live Controls"(w314) -> ()
                        n295 = call "ESA-C Get Values.vi"("Drive Connection Settings"=w316) -> ("Drive Current Values"=w315:T9)
                        n296 = local write "Drive Live Current Values"(w315) -> ()
                      }
                    }
                  }
                  frame #1 {
                    # "Snapshot"
                    n297 = Unbundle By Name(w317) -> ("Snapshot"=w320:bool)
                    n298 = case shown="True" w320 {
                      selector: w320 -> [w321 _]
                      tunnel: [w321 FALSE] -> w319
                      frame False {
                      }
                      frame True {
                        n299 = call "Video Snapshot.vi"() -> ()  [unwired: 11 in, 1 out]
                      }
                    }
                    n300 = Bundle By Name(cluster=w317, "Snapshot"=w319) -> (w318:T15)
                    n301 = local write "Drive Live Controls"(w318) -> ()
                  }
                  frame #2 {
                    n302 = property on="Read Drive" class="Bool (strict)"("Val(Sgnl)"=TRUE ("Wert (signalisierend)")) -> ()  [unwired: 2 in, 2 out]
                  }
                }
              }
            }
          }
          event "Spectrum Save": Value Change {
            n303 = event-data() -> ("NewVal"=w324:bool)  [unwired: 1 in, 4 out]
            n304 = stacked-sequence {
              tunnel: w324 -> [w325 _]
              frame #0 {
                n305 = case shown="True" w325 {
                  frame False {
                  }
                  frame True {
                    n306 = local read "Spectrum"() -> (w329:cluster{dbl[], dbl[]}[])
                    n307 = local read "CCD3500 Temperature"() -> (w333:dbl)
                    n308 = local read "ITC503 Current Values"() -> (w334:T7)
                    n309 = local read "Drive Current Values"() -> (w335:T9)
                    n310 = local read "iHR Current Values"() -> (w337:T14)
                    n311 = local read "Spectra Settings"() -> (w336:T12)
                    n312 = Index Array(array=w329, index=0 ("Index")) -> (element=w327:cluster{dbl[], dbl[]})
                    n313 = Unbundle(w327) -> (w340:dbl[], w339:dbl[])
                    n314 = Build Array(w340, w339) -> (w338:dbl[][])
                    n315 = call "Export_spectrumFileName.vi"("ITC503 Current Values"=w334, "iHR Current Values"=w337, "Spectra Settings"=w336, "Drive Current Values"=w335, "CCD3500 Temperature"=w333) -> ("Filename"=w332:string)
                    n316 = local read "Spectrum Autosave"() -> (w330:bool)
                    n317 = local read "Auto Folder"() -> (w326:path)
                    n318 = call "Export_2DtoTxt v10.2.0.vi"("Auto Folder"=w326, "Auto?"=w330, "Data (2D)"=w338, "Export Type"="Spectrum", "Filename"=w332) -> ()  [unwired: 1 in]
                  }
                }
              }
              frame #1 {
                n319 = local write "Spectrum Save"(FALSE ("Spectrum Save")) -> ()
              }
            }
          }
          event "Spectrum Load": Value Change {
            n320 = event-data() -> ("NewVal"=w342:bool)  [unwired: 1 in, 4 out]
            n321 = stacked-sequence {
              tunnel: w342 -> [w343 _]
              frame #0 {
                n322 = case shown="True" w343 {
                  frame False {
                  }
                  frame True {
                    n323 = local read "Spectrum"() -> (w346:cluster{dbl[], dbl[]}[])
                    n324 = call "Load Spectrum.vi"() -> ("Graph Cluster"=w344:cluster{dbl[], dbl[]})  [unwired: 3 in, 2 out]
                    n325 = Build Array (concatenate)(w346, w344) -> (w345:cluster{dbl[], dbl[]}[])
                    n326 = local write "Spectrum"(w345) -> ()
                  }
                }
              }
              frame #1 {
                n327 = local write "Spectrum Load"(FALSE ("Spectrum Load")) -> ()
              }
            }
          }
          event "Spectrum Autosave": Value Change {
            n328 = event-data() -> ("NewVal"=w349:bool)  [unwired: 1 in, 4 out]
            n329 = case shown="True" w349 {
              tunnel: [path "" w355] -> w348
              frame False {
              }
              frame True {
                n330 = call "File Dialog"("prompt"="Choose Save Folder") -> ("selected path"=w357:path, "cancelled"=w351:bool, "error out"=w353:errorcluster)  [unwired: 11 in, 1 out]
                n331 = call <vilib>:"Simple Error Handler.vi"("error in (no error)"=w353) -> ("error?"=w352:bool)  [unwired: 4 in, 4 out]
                n332 = Or(x=w351, y=w352) -> (x .or. y?=w354:bool)
                n333 = case shown="True" w354 {
                  tunnel: w357 -> [w358 _]
                  tunnel: [w358 path ""] -> w355
                  frame False {
                  }
                  frame True {
                    n334 = local write "Spectrum Autosave"(FALSE ("Spectrum Autosave")) -> ()
                  }
                }
              }
            }
            n335 = local write "Auto Folder"(w348) -> ()
          }
          event "Spectrum Maximize": Value Change {
            n336 = event-data() -> ("NewVal"=w361:bool)  [unwired: 1 in, 4 out]
            n337 = case shown="True" w361 {
              frame False {
                n338 = local read "Spectrum Properties"() -> (w364:cluster{"Position":T1, "Plot Area Size":T1})
                n339 = Unbundle(w364) -> ("Position"=w363:T1, "Plot Area Size"=w362:T1)
                n340 = stacked-sequence {
                  tunnel: w363 -> [_ w366]
                  tunnel: w362 -> [w365 _]
                  frame #0 {
                    n341 = property on="Spectrum" class="XYGraph (strict)"("Plot Area Size"=w365) -> ()  [unwired: 2 in, 2 out]
                  }
                  frame #1 {
                    n342 = property on="Spectrum" class="XYGraph (strict)"("Position"=w366) -> ()  [unwired: 2 in, 2 out]
                  }
                }
              }
              frame True {
                n343 = property on="Spectrum" class="XYGraph (strict)"() -> ("Bounds"=w387:T1, "Plot Area Size"=w386:T1, "Position"=w384:T22)  [unwired: 2 in, 2 out]
                n344 = Bundle("Position"=w384, "Plot Area Size"=w386) -> (w385:cluster{"Position":T22, "Plot Area Size":T1})  [unwired: 1 in]
                n345 = Unbundle By Name(w387) -> ("Width"=w391:u32, "Height"=w392:u32)
                n346 = Unbundle By Name(w386) -> ("Width"=w394:u32, "Height"=w393:u32)
                n347 = property on="Register" class="TabCtl (strict)"() -> ("Bounds"=w390:T1, "Position"=w379:T22, "Width"=w370:u32, "Height"=w369:u32)  [unwired: 2 in, 2 out]
                n348 = local write "Spectrum Properties"(w385) -> ()
                n349 = Subtract(x=w391, y=w394) -> (x-y=w383:u32)
                n350 = Subtract(x=w392, y=w393) -> (x-y=w380:u32)
                n351 = Add(x=w383, y=u32 25) -> (x+y=w382:u32)
                n352 = Add(x=w380, y=u32 70) -> (x+y=w381:u32)
                n353 = Subtract(x=w370, y=w382) -> (x-y=w389:u32)
                n354 = Subtract(x=w369, y=w381) -> (x-y=w388:u32)
                n355 = Bundle By Name(cluster=w390, "Width"=w389, "Height"=w388) -> (w367:T1)
                n356 = Unbundle By Name(w379) -> ("Left"=w378:i32, "Top"=w375:i32)
                n357 = Add(x=w378, y=20) -> (x+y=w377:i32)
                n358 = Add(x=w375, y=50) -> (x+y=w376:i32)
                n359 = Bundle By Name(cluster=w379, "Left"=w377, "Top"=w376) -> (w368:T22)
                n360 = stacked-sequence {
                  tunnel: w368 -> [w395 _]
                  tunnel: w367 -> [_ w396]
                  frame #0 {
                    n361 = property on="Spectrum" class="XYGraph (strict)"("Position"=w395) -> ()  [unwired: 2 in, 2 out]
                  }
                  frame #1 {
                    n362 = property on="Spectrum" class="XYGraph (strict)"("Plot Area Size"=w396) -> ()  [unwired: 2 in, 2 out]
                  }
                }
              }
            }
          }
          event "Mapping Start": Value Change {
            n363 = event-data() -> ("NewVal"=w397:bool)  [unwired: 1 in, 4 out]
            n364 = case shown="True" w397 {
              frame False {
              }
              frame True {
                n365 = stacked-sequence {
                  frame #0 {
                    n366 = property on="Measurement Running" class="Bool (strict)"("Blinking"=TRUE ("Blinkend")) -> ()  [unwired: 2 in, 2 out]
                  }
                  frame #1 {
                    w413 = FALSE ("Simulate Drive")
                    n367 = local read "CCD3500V Connection"() -> (w409:T2)
                    n368 = local read "CCD3500 Temperature"() -> (w411:dbl)
                    n369 = local read "ITC503 Current Values"() -> (w406:T7)
                    n370 = local read "Drive Current Values"() -> (w404:T9)
                    n371 = local read "iHR Current Values"() -> (w405:T14)
                    n372 = local read "Wavelengths (nm)"() -> (w407:dbl[])
                    n373 = local read "Drive Connection"() -> (w408:T10)
                    n374 = local read "CCD3500V Status"() -> (w400:bool)
                    n375 = local read "Spectra Settings"() -> (w410:T12)
                    n376 = local read "Drive Status"() -> (w402:bool)
                    n377 = Not(x=w402) -> (.not. x?=w401:bool)
                    n378 = Not(x=w400) -> (.not. x?=w399:bool)
                    n379 = Bundle By Name(cluster=T20 {"CCD3000 Connection"={"Comm Interface"=1, "BUS"=0, "Address"=5, "Com Port"=1}, "Drive Connection Settings"={"Objective GPIB-Port"=4, "Stage GPIB-Port"=4, "Drive Selector"=0, "Drive Velocity (V/s)"=5.0}, "ITC503 Current Values"={"ITC503 Heater"=0.0, "ITC503 Temperature"=0.0, "ITC503 P"=0.0, "ITC503 I"=0.0, "ITC503 D"=0.0, "ITC503 Setpoint"=0.0, "ITC503 Gradient"=0.0, "ITC503 Heater Auto"=FALSE, "ITC503 PID Auto"=FALSE}, "Wavelengths (nm)"=[], "Drive Current Values"={"Voltages"={"Drive X Voltage"=0.0, "Drive Y Voltage"=0.0, "Drive Z Voltage"=0.0}, "Position"={"Drive X Position"=0.0, "Drive Y Position"=0.0, "Drive Z Position"=0.0}}, "iHR Current Values"={"iHR 550 Front Entrance"=0.0, "iHR550 Side Exit"=0.0, "iHR550 Wavelength"=897.9988, "iHR550 Exit Mirror"=2, "iHR550 Grating"="1", "Grating Index"=1}, "Spectra Settings"={"Integration Time"=1.0, "Repetitions"=1, "Mapping Spectra"=TRUE}, "CCD3500 Temperature"=0.0, "Simulate Drive 2"=FALSE, "Simulate Spectra 2"=FALSE} ("Input Parameters"), "CCD3000 Connection"=w409, "Drive Connection Settings"=w408, "ITC503 Current Values"=w406, "Wavelengths (nm)"=w407, "Drive Current Values"=w404, "iHR Current Values"=w405, "Spectra Settings"=w410, "CCD3500 Temperature"=w411, "Simulate Drive 2"=w401, "Simulate Spectra 2"=w399) -> (w412:T20)
                    n380 = call "Mapping v10.2.0.vi"("Simulate Spectra"=w413, "Simulate Drive"=w413, "Input Parameters"=w412) -> ()  [unwired: 9 in]
                  }
                  frame #2 {
                    # "reinitialize CCD after mapping"
                    n381 = local read "CCD3500V Connection"() -> (w414:T2)
                    n382 = local read "Spectra Settings"() -> (w416:T12)
                    n383 = call "CCD3000 Prepare Acquisition.vi"("Mapping Spectra Settings"=w416, "Comm Params"=w414) -> ()  [unwired: 4 in]
                    n384 = Unbundle By Name(w416) -> ("Integration Time"=w415:dbl)
                    n385 = local write "Int. Time Temp"(w415) -> ()
                  }
                  frame #3 {
                    w417 = FALSE ("Mapping Start")
                    n386 = local write "Mapping Start"(w417) -> ()
                    n387 = property on="Measurement Running" class="Bool (strict)"("Blinking"=w417) -> ()  [unwired: 2 in, 2 out]
                  }
                }
              }
            }
          }
        }
      }
    }
    frame #3 {
      # "Close Connections"
      n388 = control-ref of="Dieses VI"() -> (w418:refnum<vi>)
      n389 = invoke class="VI" method="Default Vals.Reinit All"(reference=w418) -> ()  [unwired: 2 in, 3 out]
    }
  }
